vi "InitMessageStartBuffer.vi"(8 "error in (no error)":errorcluster, 11 "TCP_Client in":refnum<class "TCP_Client.lvclass">) -> (0 "error out":errorcluster, 3 "TCP_Client out":refnum<class "TCP_Client.lvclass">)   [LabVIEW 2023, in "TCP_Client.lvlib" / "TCP_Client.lvclass"]
uses:
  TCP_Client.lvclass
  TCP_Client.lvclass/TCP_Client.ctl
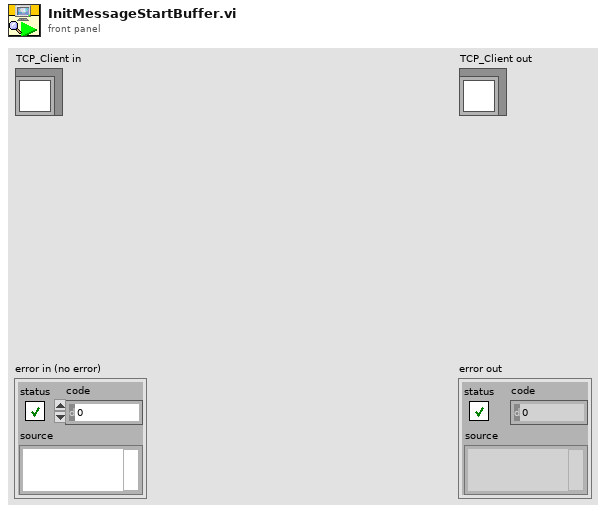
[diagram p1: front panel]
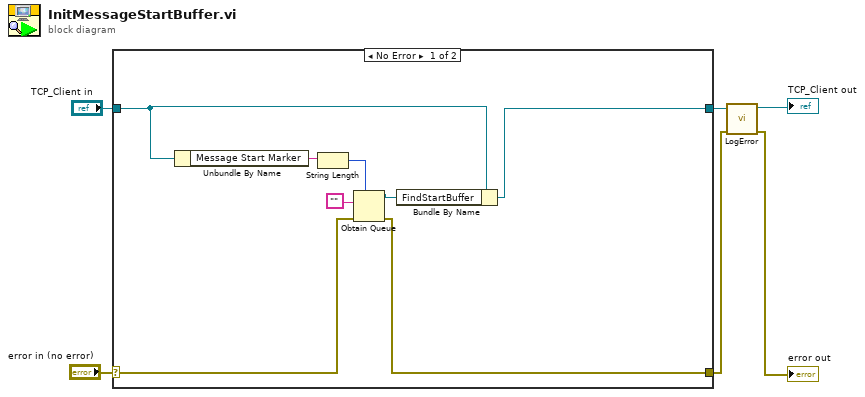
[diagram p0: block diagram]
diagram:
  n1 = case shown="No Error" "error in (no error)" {
    selector: "error in (no error)" -> [w11 w16]
    tunnel: [w10 w16] -> w2
    tunnel: [w7 w15] -> w4
    tunnel: "TCP_Client in" -> [w9 w15]
    frame No Error {
      n2 = Unbundle By Name(w9) -> ("Message Start Marker"=w14:string)
      n3 = String Length(string=w14) -> (length=w12:i32)
      n4 = Obtain Queue(max queue size (-1, unlimited)=w12, element data type="", error in (no error)=w11) -> (queue out=w8:refnum<queue>, error out=w10:errorcluster)  [unwired: 2 in, 1 out]
      n5 = Bundle By Name(cluster=w9, "FindStartBuffer"=w8) -> (w7:refnum<class "TCP_Client.lvclass">)
    }
    frame Error {
    }
  }
  n6 = call "LogError.vi"("error in (no error)"=w2, "TCP_Client in"=w4) -> ("error out"=→"error out":errorcluster, "TCP_Client out"=→"TCP_Client out":refnum<class "TCP_Client.lvclass">)  [unwired: 8 in]
